vi "AddAdditionalFields.vi"(8 "error in (no error)":errorcluster, 10 "Menu":refnum<class "MGI_Menu.lvclass">, 11 "MenuStripItem in":refnum<class "MGI_MenuStripItem.lvclass">) -> (0 "error out":errorcluster, 2 "Menu out":refnum<class "MGI_Menu.lvclass">, 3 "MenuStripItem out":refnum<class "MGI_MenuStripItem.lvclass">)   [LabVIEW 2016, in "MGI_MenuStripItem.lvclass"]
doc: "No-op for a standard Menu Item. Used by children classes to add additional fields (Like shortcuts, etc)\n\nAuthored by Derek E. Trepanier\nsupport@mooregoodideas.com\nwww.mooregoodideas.com\n\nCopyright (c) 2012, Moore Good Ideas, Inc.\n\nAll rights reserved.\n\nRedistribution and use in source and binary forms, with or without modification, are permitted provided that the following conditions are met:\n\n * Redistributions of source code must retain the above copyright notice, this list of conditions and the following disclaimer.\n * Redistributions in binary form must reproduce the above copyright notice, this list of conditions and the following disclaimer in the documentation and/or other materials provided with the distribution.\n * Neither the name of Moore Good Ideas, Inc. nor the names of its contributors may be used to endorse or promote products derived from this software without specific prior written permission.\n\nTHIS SOFTWARE IS PROVIDED BY THE COPYRIGHT HOLDERS AND CONTRIBUTORS \"AS IS\" AND ANY EXPRESS OR IMPLIED WARRANTIES, INCLUDING, BUT NOT LIMITED TO, THE IMPLIED WARRANTIES OF MERCHANTABILITY AND FITNESS FOR A PARTICULAR PURPOSE ARE DISCLAIMED. IN NO EVENT SHALL THE COPYRIGHT OWNER OR CONTRIBUTORS BE LIABLE FOR ANY DIRECT, INDIRECT, INCIDENTAL, SPECIAL, EXEMPLARY, OR CONSEQUENTIAL DAMAGES (INCLUDING, BUT NOT LIMITED TO, PROCUREMENT OF SUBSTITUTE GOODS OR SERVICES; LOSS OF USE, DATA, OR PROFITS; OR BUSINESS INTERRUPTION) HOWEVER CAUSED AND ON ANY THEORY OF LIABILITY, WHETHER IN CONTRACT, STRICT LIABILITY, OR TORT (INCLUDING NEGLIGENCE OR OTHERWISE) ARISING IN ANY WAY OUT OF THE USE OF THIS SOFTWARE, EVEN IF ADVISED OF THE POSSIBILITY OF SUCH DAMAGE."
uses:
  <userlib>/_MGI/Menu Building/MenuItem/MenuStripItem/MGI_MenuStripItem.lvclass
  C:/Program Files (x86)/National Instruments/LabVIEW 2016/user.lib/_MGI/Menu Building/MenuItem/MGI_MenuItem.lvclass
  <userlib>/_MGI/Menu Building/MenuTypes/MGI_Menu.lvclass
  <userlib>/_MGI/Menu Building/MenuTypes/MenuStrip/MGI_MenuStrip.lvclass
  C:/Program Files (x86)/National Instruments/LabVIEW 2016/user.lib/_MGI/Menu Building/MenuTypes/MGI_Menu.lvclass
  <userlib>/_MGI/Menu Building/MenuItem/MenuStripItem/MGI_MenuStripItem.lvclass/MGI_MenuStripItem.ctl
  System.Drawing
  System.Windows.Forms
  <userlib>/_MGI/Menu Building/MenuItem/Read Full Tag.vi
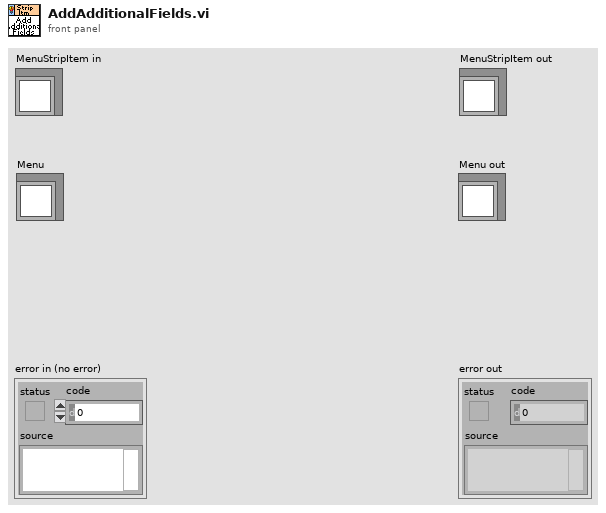
[diagram p1: front panel]
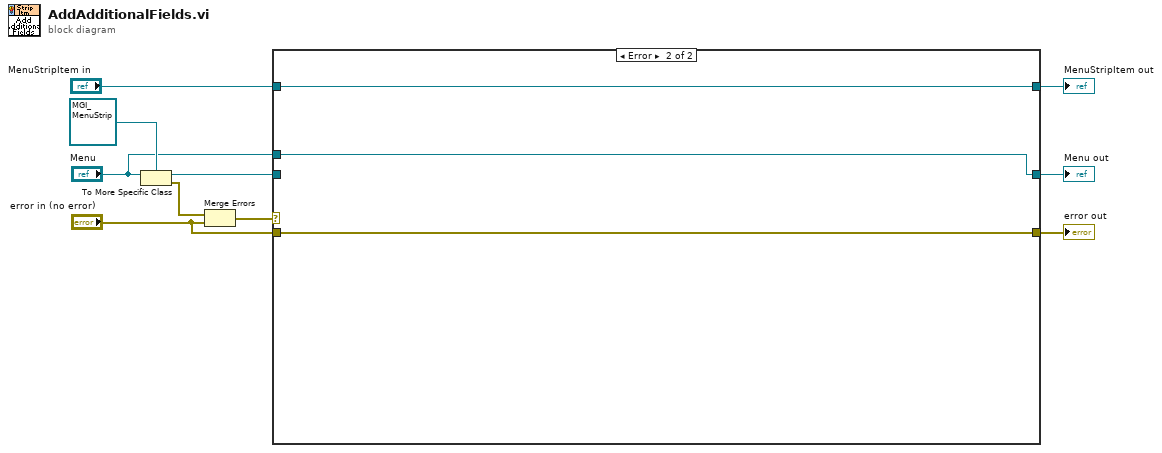
[diagram p0: block diagram]
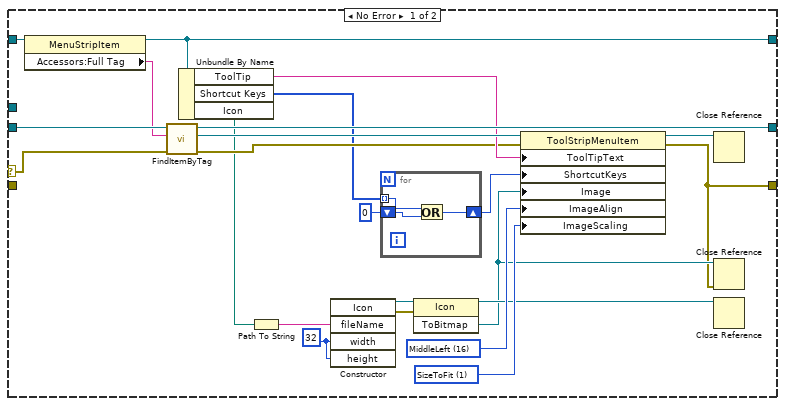
[diagram p2: hidden frame]
diagram:
  n1 = To More Specific Class(target class=refnum<class "MGI_MenuStrip.lvclass"> refnum ("MenuStrip.lvclass"), reference="Menu") -> (specific class reference=w6:refnum<class "MGI_MenuStrip.lvclass">, error out=w3:errorcluster)  [unwired: 1 in]
  n2 = Merge Errors(w3, "error in (no error)") -> (w4:errorcluster)
  n3 = case shown="Error" w4 {
    selector: w4 -> [w30 _]
    tunnel: [w11 w38] -> w10
    tunnel: [w29 w37] -> w9
    tunnel: w6 -> [w33 _]
    tunnel: [w27 w39] -> w8
    tunnel: "MenuStripItem in" -> [w32 w39]
    tunnel: "error in (no error)" -> [_ w38]
    tunnel: "Menu" -> [_ w37]
    frame No Error {
      w17 = 1 items=["None", "SizeToFit"] ("ImageScaling")
      w18 = 16 items=["TopLeft"=1, "TopCenter"=2, "TopRight"=4, "MiddleLeft"=16, "MiddleCenter"=32, "MiddleRight"=64, "BottomLeft"=256, "BottomCenter"=512, "BottomRight"=1024] ("ImageAlign")
      w21 = 32 ("width")
      n4 = property class="MenuStripItem"(reference=w32) -> (reference out=w27:refnum<class "MGI_MenuStripItem.lvclass">, "Accessors:Full Tag"=w31:string)  [unwired: 1 in, 1 out]
      n5 = call <userlib>:"FindItemByTag.vi"("error in (no error)"=w30, "Tag"=w31, "MenuStrip in"=w33) -> ("error out"=w25:errorcluster, "Tool Strip Menu Item"=w28:refnum<k24>, "MenuStrip out"=w29:refnum<class "MGI_MenuStrip.lvclass">)  [unwired: 6 in]
      n6 = Unbundle By Name(w27) -> ("ToolTip"=w26:string, "Shortcut Keys"=w24:i32[], "Icon"=w16:path)
      n7 = Path To String(path=w16) -> (string=w15:string)
      n8 = constructor class="Icon"("fileName"=w15, "width"=w21, "height"=w21) -> (reference out=w19:refnum<k24>, error out=w20:errorcluster)  [unwired: 3 in, 4 out]
      n9 = for {
        tunnel: w24 -> [w36] mode=indexing
        shift-right: [w35] -> w22
        shift-left: 0 -> [w34]
        n10 = Or(x=w36, y=w34) -> (x .or. y?=w35:i32)
      }
      n11 = invoke class="Icon" method="ToBitmap"(reference=w19, error in=w20) -> (reference out=w13:refnum<k24>, "ToBitmap"=w12:refnum<k24>)  [unwired: 1 in, 1 out]
      n12 = property class="ToolStripMenuItem"(reference=w28, error in=w25, "ToolTipText"=w26, "ShortcutKeys"=w22, "Image"=w12, "ImageAlign"=w18, "ImageScaling"=w17) -> (reference out=w14:refnum<k24>, error out=w11:errorcluster)
      n13 = Close Reference(reference=w14) -> ()  [unwired: 1 in, 1 out]
      n14 = Close Reference(reference=w12, error in (no error)=w11) -> ()  [unwired: 1 out]
      n15 = Close Reference(reference=w13) -> ()  [unwired: 1 in, 1 out]
    }
    frame Error {
    }
  }
  "error out" <- w10
  "MenuStripItem out" <- w8
  "Menu out" <- w9
